vi "Preview.vi"(8 "error in (no error)":errorcluster, 11 "RTM View in":refnum<class "RTM View.lvclass">) -> (0 "error out":errorcluster, 3 "RTM View out":refnum<class "RTM View.lvclass">)   [LabVIEW 2013, in "SET Project Editor.lvlib" / "RTM View.lvclass"]
uses:
  RTM View.lvclass
  RTM View.lvclass/RTM View.ctl
  SET Project Data/Menu Class/Read Languages.vi
  SET Project Editor.lvlib
  SET Project Data/Menu Class/Menu Data.lvclass
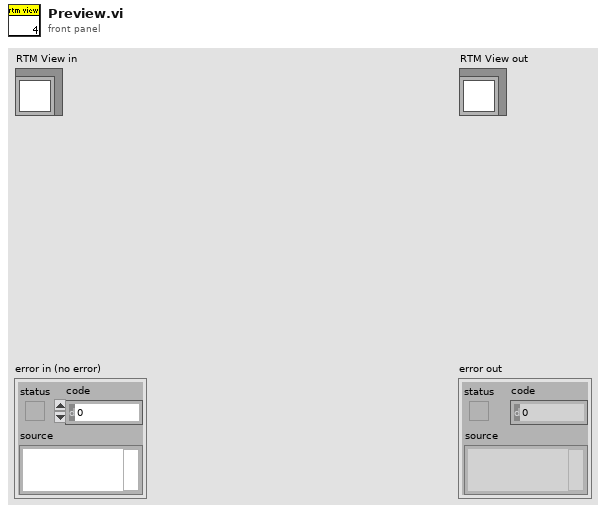
[diagram p1: front panel]
types:
  T1 = typedef "SET Resource File.lvlib/ResFile Lang Entry.ctl" = cluster{"Tag":string, "Name":string, "Code Page":u16}
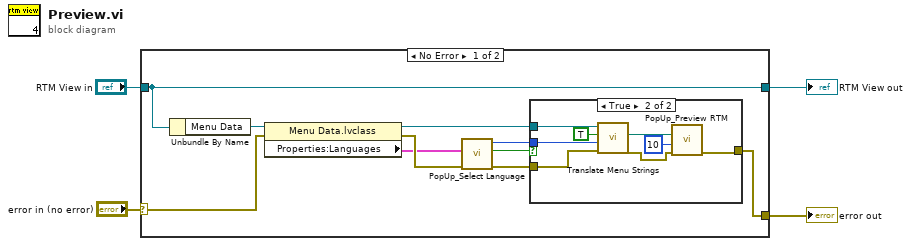
[diagram p0: block diagram]
diagram:
  n1 = case shown="No Error" "error in (no error)" {
    selector: "error in (no error)" -> [w11 w24]
    tunnel: "RTM View in" -> [w5 w25]
    tunnel: [w6 w24] -> w2
    tunnel: [w5 w25] -> w1
    frame No Error {
      n2 = Unbundle By Name(w5) -> ("Menu Data"=w12:refnum<class "Menu Data.lvclass">)
      n3 = property class="Menu Data.lvclass"(reference=w12, error in=w11) -> (reference out=w8:refnum<class "Menu Data.lvclass">, error out=w14:errorcluster, "Properties:Languages"=w13:T1[])
      n4 = call "PopUp_Select Language.vi"("error in (no error)"=w14, "Languages"=w13) -> ("error out"=w7:errorcluster, "OK Pressed?"=w10:bool, "LangIndex"=w9:i32)  [unwired: 7 in]
      n5 = case shown="True" w10 {
        tunnel: w9 -> [_ w22]
        tunnel: w8 -> [_ w23]
        tunnel: w7 -> [w15 w21]
        tunnel: [w15 w16] -> w6
        frame False {
        }
        frame True {
          n6 = call "Translate Menu Strings.vi"("error in (no error)"=w21, "Language Index (0)"=w22, "Preview?"=TRUE, "Menu Data in"=w23) -> ("error out"=w17:errorcluster, "Preview Path out"=w19:path)  [unwired: 5 in, 1 out]
          n7 = call "PopUp_Preview RTM.vi"("error in (no error)"=w17, "Timeout"=10, "RTM Path"=w19) -> ("error out"=w16:errorcluster)  [unwired: 8 in]
        }
      }
    }
    frame Error {
    }
  }
  "error out" <- w2
  "RTM View out" <- w1
